vi "test_interp_extrap.vi"() -> ()   [LabVIEW 2018]
uses:
  <vilib>/Simulation/Scripting/Companion Diagram/SimConfigNode/SimParams.ctl
  <vilib>/Simulation/Scripting/Companion Diagram/SimConfigNode/_simSolvers.ctl
  <vilib>/Simulation/Implementation/Shared/SIMSCR Execution Mode.ctl
  <vilib>/Simulation/Param Hierarchy/Typedefs/SIMPH Param Control Actions.ctl
  <vilib>/Analysis/1siggen.llb/Ramp Pattern by Samples.vi
  <vilib>/Simulation/Implementation/Shared/NILVSim_ParamChanged.vi
  <vilib>/Simulation/Implementation/Shared/NILVSIM_BeginStep.vi
  <vilib>/Simulation/LookUpTables/Implementation/NILVSim LUT 1D.llb/SIM LUT 1D (scalar).vi
  <vilib>/Simulation/Implementation/Shared/NILVSim_Manager.vi
  <vilib>/Utility/error.llb/Clear Errors.vi
  <vilib>/Simulation/Implementation/Shared/NILVSim_FinalizeModel.vi
  <vilib>/Utility/file.llb/Read Delimited Spreadsheet (DBL).vi
  <vilib>/Simulation/Implementation/Shared/SIM Unbundle Sim Info.vi
  <vilib>/Simulation/Implementation/Shared/NILVSim_Initialize.vi
  <vilib>/Simulation/Utility/Implementation/NILVSim Get Time and IsAcceptedStep.vi
  <vilib>/Simulation/Implementation/Shared/SIMSH Read Queue.vi
  <vilib>/Simulation/Implementation/Shared/NILVSim_GetModelError.vi
  <vilib>/Simulation/Implementation/Shared/SIM Bundle Sim Info.vi
  <vilib>/Simulation/Scripting/Companion Diagram/SimConfigNode/SimDog.xnode
  <vilib>/Simulation/Implementation/XNodeFramework/SimXNode/SimX.xnode
  <vilib>/Analysis/NI_AALBase.lvlib
  <vilib>/Simulation/Implementation/Shared/NI_SIM_Implementation.lvlib
panel:
  in  "stop":bool
  out "Theta_d: Interp Results":dbl
  out "Theta_d: LUT Results":dbl
  out "K: Interp Results":dbl
  out "K: LUT Results":dbl
  in  "Current gait %":dbl
  out "Gait %: Interp Results":dbl
  out "Gait %: LUT Results":dbl
  in  "Current Phi":dbl
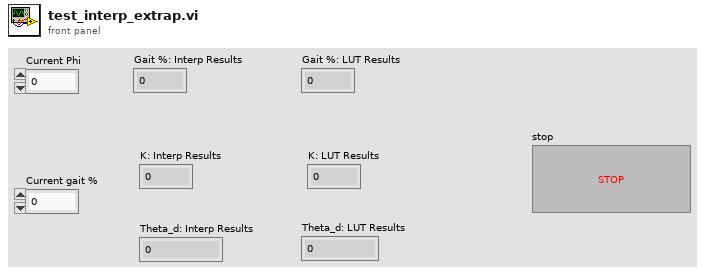
[diagram p1: front panel]
types:
  T1 = enum16{"Interpolate/Extrapolate", "Interpolate", "Nearest", "Below", "Above"}
  T2 = typedef "SIMSCR Execution Mode.ctl" = enum16{"Simulate to Completion", "Single Time-Step Simulation (Fixed Step Only)"}
  T3 = typedef "SIMPH Param Control Actions.ctl" = enum16{"get params", "set params"}
  T4 = typedef "SimParams.ctl" = cluster{"Initial Time (s)":dbl, "Final Time (s)":dbl, "Step Size (s)":dbl, "ODE Solver":T5, "Minimum Step Size (s)":dbl, "Maximum Step Size (s)":dbl, "Relative Tolerance":dbl, "Absolute Tolerance":dbl, "Software Timing":bool, "Initial Step Size (s)":dbl, "Automatic Fixed Step Size?":bool, "Automatic Discrete Step Size?":bool, "Discrete Step Size (s)":dbl, "Calculate using Time Step":bool, "Solver Wired?":bool, "Prev.Frm.Expected End":u64, "Prev.Frm.Actual End":u64, "Prev.Frm.Finished Late?":bool, "Prev.Iter.Expected End":u64, "Prev.Iter.Actual End":u64, "Prev.Iter.Finished Late?":bool, "Expected Iteration Start":u64, "Actual Iteration Start":u64, "Expected Frame Start":u64, "Actual Frame Start":u64, "Source Name":string, "Name":string, "Period":i64, "Deadline":i64, "Offset":i64, "Start":i64, "Priority":i32, "Timeout":i32, "Processor":i32, "Mode":enum32{"No Change", "Process missed periods, maintain original phase", "Discard missed periods, maintain original phase", "Process missed periods, ignore original phase", "Discard missed periods, ignore original phase"}, "Wakeup reason":enum32{"Normal", "Aborted", "Asynchronous wakeup", "Timing source error", "Timed loop error", "Timeout"}, "Error":errorcluster, "Source Type":string, "Secondary Source Type":string, "Global End Time":u64, "Global Start Time":u64, "Full Solver Reset":bool, "Execution Mode":T2, "Nan/Inf Check":bool, "Custom Solver Library":string, "Solver Is Variable":bool, "custom solver name":string, "Signal Collection Decimation":u32}
  T5 = typedef "_simSolvers.ctl" = enum16{"Runge-Kutta 1 (Euler)", "Runge-Kutta 2", "Runge-Kutta 3", "Runge-Kutta 4", "Runge-Kutta 23 (variable)", "Runge-Kutta 45 (variable)", "BDF (variable)", "Adams-Moulton (variable)", "Rosenbrock (variable)", "Discrete States Only", "SDIRK 4 (variable)", "Radau 5 (variable)", "Radau 9 (variable)", "Radau 13 (variable)", "Radau [Variable Order] (variable)", "Gear's Method (variable)", "Linearizer", "State Query", "Trim Eval", "Custom Solver"}
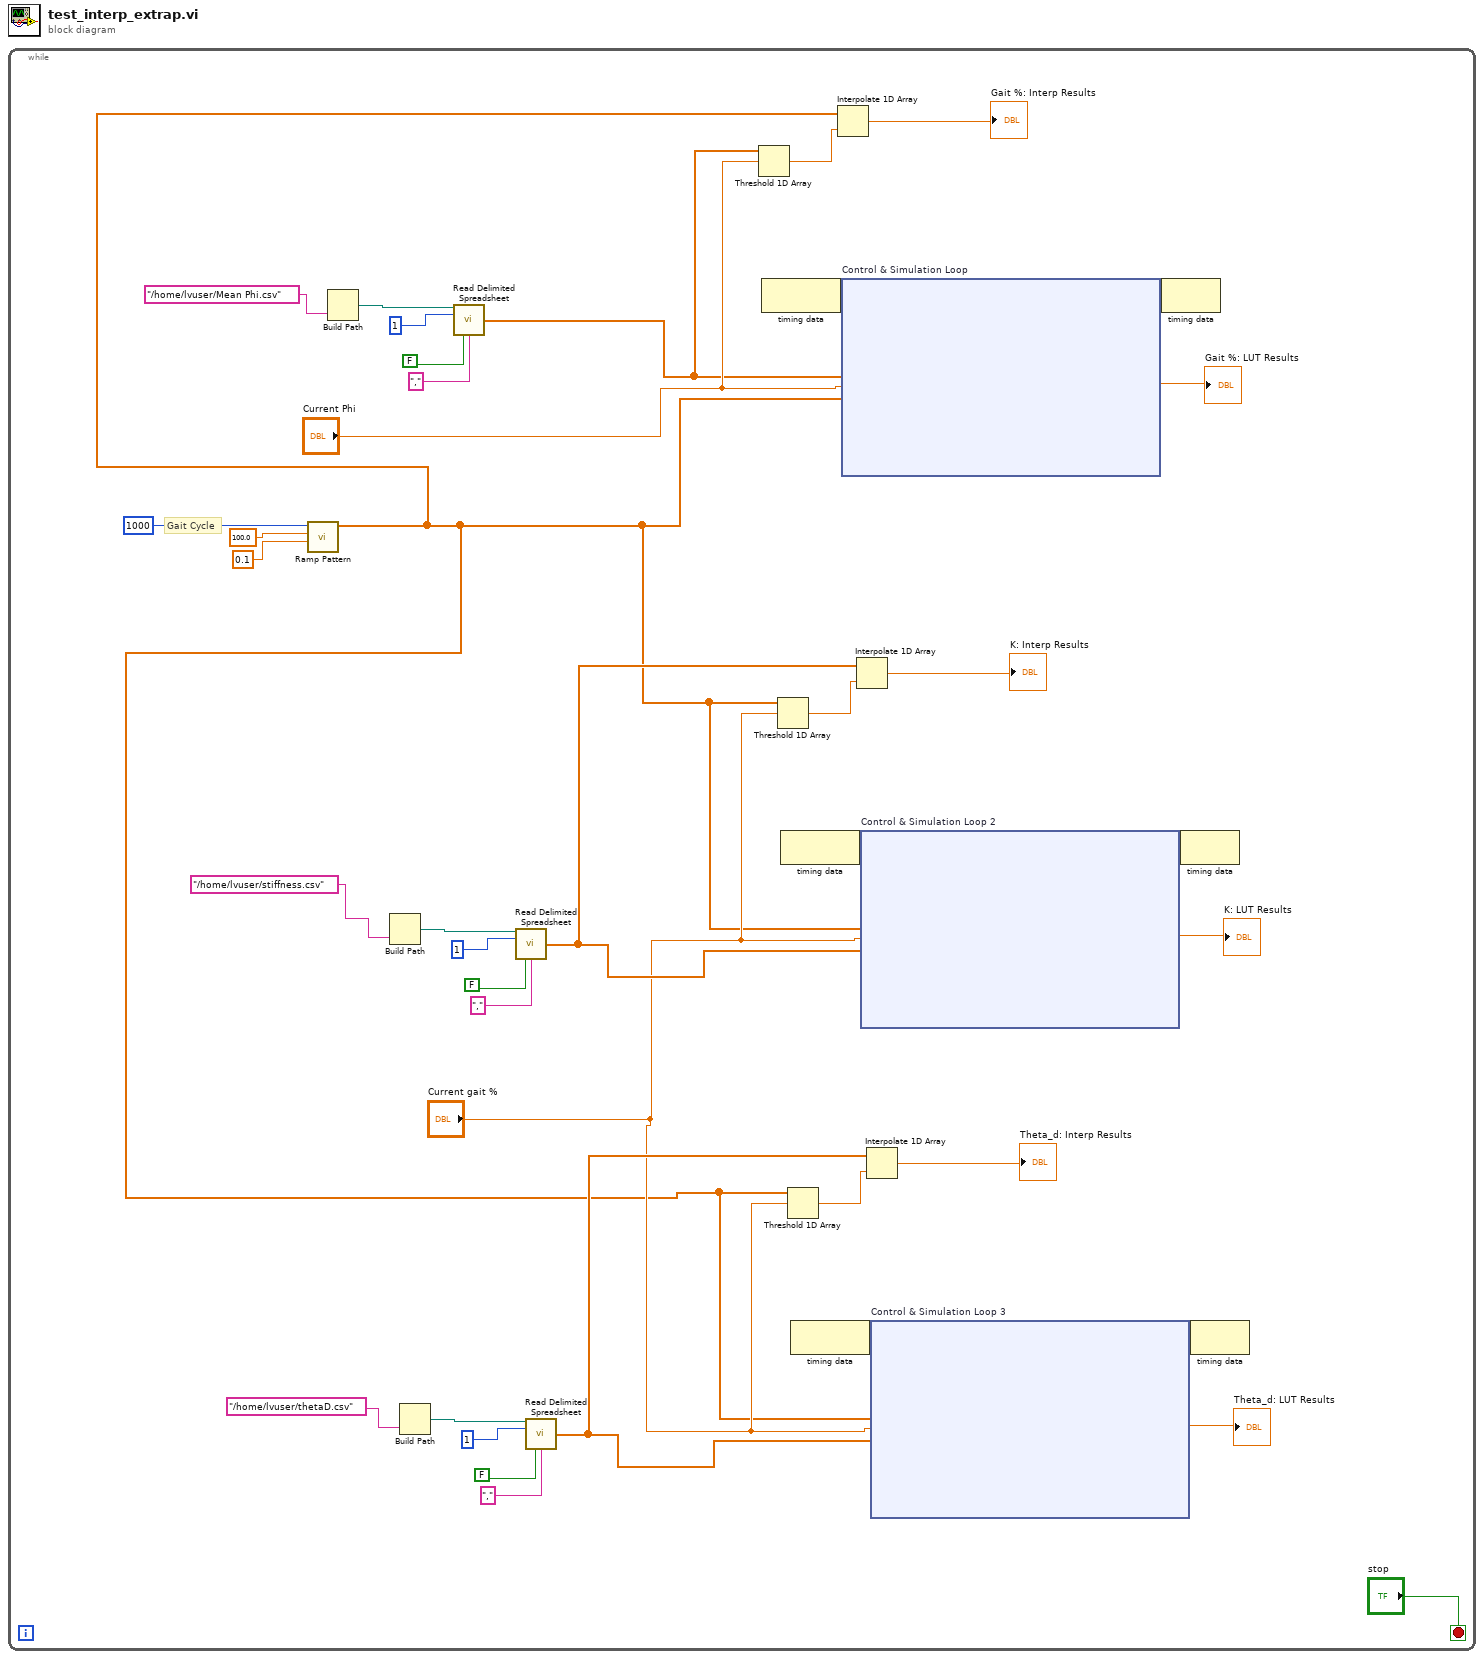
[diagram p0: block diagram]
diagram:
  n1 = while {
    stop <- "stop" stop-if-true
    # "Gait Cycle"
    n2 = call-poly <vilib>:"Ramp Pattern.vi"("start"=0.1, "end"=100.0, "samples"=1000) -> ("Ramp Pattern"=w2:dbl[])  [unwired: 7 in, 1 out]
    n3 = Build Path(name or relative path="/home/lvuser/Mean Phi.csv") -> (appended path=w28:path)  [unwired: 1 in]
    n4 = Build Path(name or relative path="/home/lvuser/stiffness.csv") -> (appended path=w15:path)  [unwired: 1 in]
    n5 = Build Path(name or relative path="/home/lvuser/thetaD.csv") -> (appended path=w6:path)  [unwired: 1 in]
    n6 = call-poly <vilib>:"Read Delimited Spreadsheet.vi"("file path (dialog if empty)"=w28, "number of rows (all:-1)"=1, "transpose? (F)"=FALSE, "delimiter (\\t)"="," ("delimiter (\\t)")) -> ("first row"=w23:dbl[])  [unwired: 6 in, 5 out]
    n7 = call-poly <vilib>:"Read Delimited Spreadsheet.vi"("file path (dialog if empty)"=w15, "number of rows (all:-1)"=1, "transpose? (F)"=FALSE, "delimiter (\\t)"="," ("delimiter (\\t)")) -> ("first row"=w13:dbl[])  [unwired: 6 in, 5 out]
    n8 = call-poly <vilib>:"Read Delimited Spreadsheet.vi"("file path (dialog if empty)"=w6, "number of rows (all:-1)"=1, "transpose? (F)"=FALSE, "delimiter (\\t)"="," ("delimiter (\\t)")) -> ("first row"=w5:dbl[])  [unwired: 6 in, 5 out]
    n9 = Threshold 1D Array(2:"Current Phi", 3:w23) -> (0:w26:dbl)  [unwired: 1 in]
    n10 = node-c288() -> (w40:variant)  [unwired: 1 in]
    n11 = Threshold 1D Array(2:"Current gait %", 3:w2) -> (0:w20:dbl)  [unwired: 1 in]
    n12 = node-c288() -> (w38:variant)  [unwired: 1 in]
    n13 = Threshold 1D Array(2:"Current gait %", 3:w2) -> (0:w11:dbl)  [unwired: 1 in]
    n14 = node-c288() -> (w36:variant)  [unwired: 1 in]
    n15 = Interpolate 1D Array(1:w26, 2:w2) -> (0:→"Gait %: Interp Results":dbl)
    n16 = node-c254 "Control & Simulation Loop"(w40, w2, w23, "Current Phi") -> (w39:variant, →"Gait %: LUT Results":dbl)  [unwired: 1 out]
    n17 = Interpolate 1D Array(1:w20, 2:w13) -> (0:→"K: Interp Results":dbl)
    n18 = node-c254 "Control & Simulation Loop 2"(w38, w13, w2, "Current gait %") -> (w37:variant, →"K: LUT Results":dbl)  [unwired: 1 out]
    n19 = Interpolate 1D Array(1:w11, 2:w5) -> (0:→"Theta_d: Interp Results":dbl)
    n20 = node-c254 "Control & Simulation Loop 3"(w36, w5, w2, "Current gait %") -> (w35:variant, →"Theta_d: LUT Results":dbl)  [unwired: 1 out]
    n21 = node-c288(w39) -> ()  [unwired: 1 out]
    n22 = node-c288(w37) -> ()  [unwired: 1 out]
    n23 = node-c288(w35) -> ()  [unwired: 1 out]
  }
